vi "sinewave_generator_simulation_demoinfocom.vi"() -> ()   [LabVIEW 2021]
uses:
  <vilib>/addons/Modulation/Analog/controls/Complex Data Waveform.ctl
  <vilib>/Analysis/1siggen.llb/Ramp Pattern by Samples.vi
  system stop.vi
  <vilib>/measure/maspectr.llb/FFT Power Spectrum and PSD for 1 Chan (CDB).vi
  <vilib>/addons/Modulation/niAMT.lvlib
  <vilib>/Analysis/NI_AALBase.lvlib
  <vilib>/measure/NI_MAPro.lvlib
panel:
  out "Waveform Graph":cluster{"f0":dbl, "df":dbl, "magnitude":dbl[]}(graph)
  in  "Sampling Rate":dbl
  in  "duration":dbl
  in  "Frequency":dbl format="%#_13g"
  in  "stop":bool
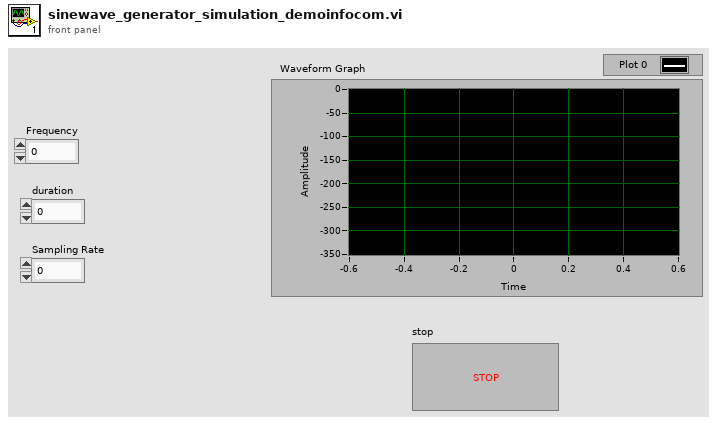
[diagram p1: front panel]
types:
  T1 = typedef "niAMT.lvlib/Complex Data Waveform.ctl" = cluster{"t0":dbl, "dt":dbl, "Y":cdb[]}
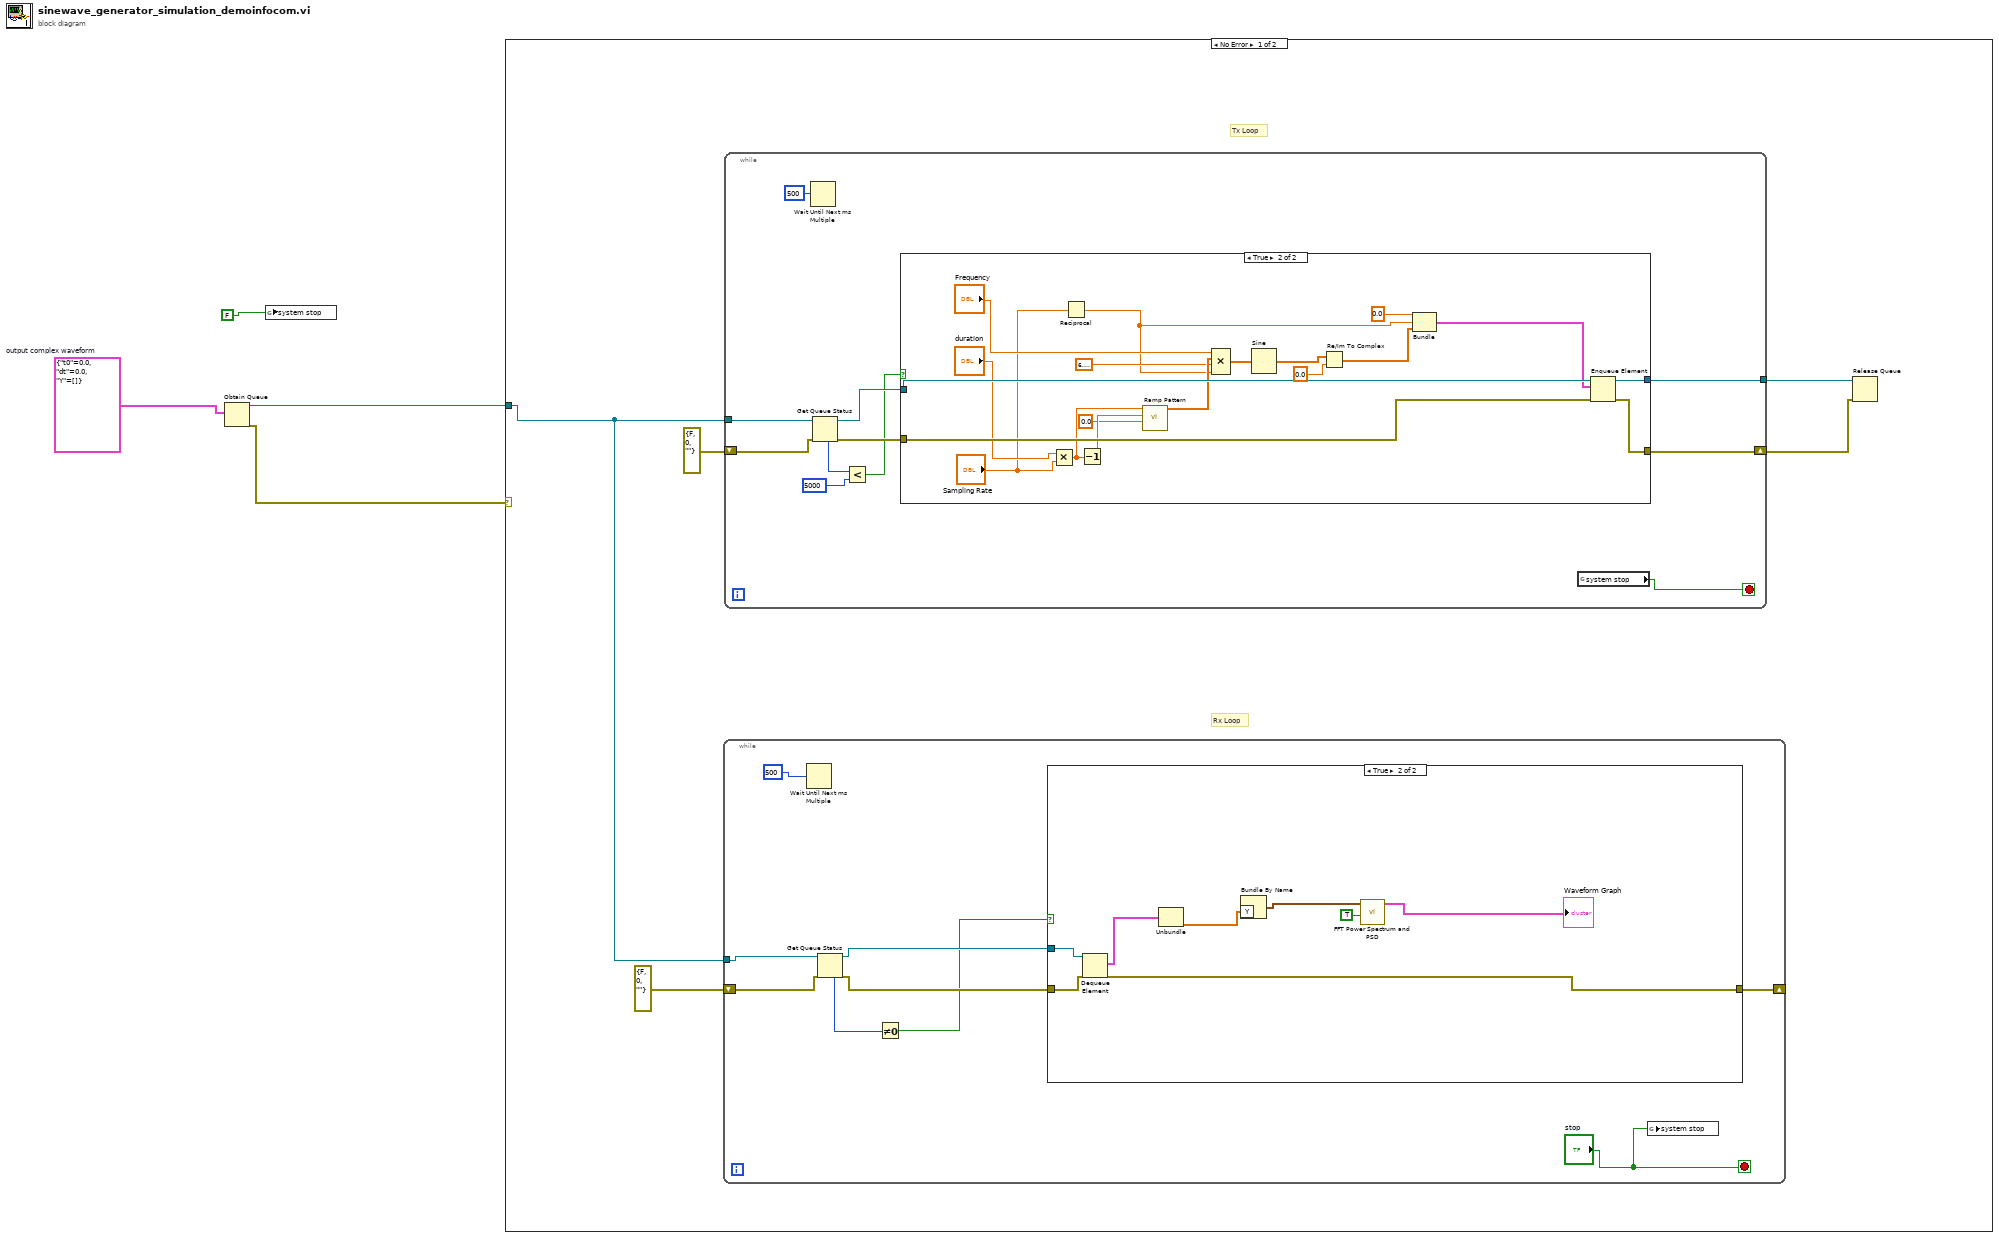
[diagram p0: block diagram]
diagram:
  w1 = T1 {"t0"=0.0, "dt"=0.0, "Y"=[]}  # output complex waveform
  n1 = Obtain Queue(element data type=w1) -> (queue out=w3:refnum<queue>, error out=w2:errorcluster)  [unwired: 4 in, 1 out]
  n2 = global write "system stop.vi" "system stop"(FALSE) -> ()
  n3 = case shown="No Error" w2 {
    tunnel: w3 -> [w8 _]
    frame No Error {
      # "Rx Loop"
      # "Tx Loop"
      n4 = while {
        tunnel: w8 -> [w17]
        shift-right: [w13] -> _
        shift-left: errorcluster {"status"=FALSE, "code"=0, "source"=""} ("error in (no error)") -> [w15]
        stop <- "stop" stop-if-true
        n5 = Wait Until Next ms Multiple(millisecond multiple=500) -> ()  [unwired: 1 out]
        n6 = Get Queue Status(queue=w17, error in (no error)=w15) -> (queue out=w16:refnum<queue>, error out=w14:errorcluster, # elements in queue=w12:i32)  [unwired: 1 in, 5 out]
        n7 = Not Equal To 0?(x=w12) -> (x != 0?=w11:bool)
        n8 = case shown="True" w11 {
          tunnel: w16 -> [_ w27]
          tunnel: w14 -> [w19 w26]
          tunnel: [w19 w25] -> w13
          frame False {
          }
          frame True {
            n9 = Dequeue Element(queue=w27, error in (no error)=w26) -> (element=w24:T1, error out=w25:errorcluster)  [unwired: 1 in, 2 out]
            n10 = Unbundle(w24) -> ("Y"=w23:cdb[])  [unwired: 2 out]
            n11 = Bundle By Name("Y"=w23) -> (w21:waveform(cdb))  [unwired: 1 in]
            n12 = call-poly <vilib>:"FFT Power Spectrum and PSD.vi"("dB On (F)"=TRUE, "time signal"=w21) -> ("Power Spectrum / PSD"=→"Waveform Graph":cluster{"f0":dbl, "df":dbl, "magnitude":dbl[]})  [unwired: 6 in, 3 out]
          }
        }
        n13 = global write "system stop.vi" "system stop"("stop") -> ()
      }
      n14 = while {
        tunnel: w8 -> [w37]
        shift-right: [w33] -> w5
        shift-left: errorcluster {"status"=FALSE, "code"=0, "source"=""} ("error in (no error)") -> [w36]
        tunnel: [w29] -> w6
        stop <- w38 stop-if-true
        n15 = Wait Until Next ms Multiple(millisecond multiple=500) -> ()  [unwired: 1 out]
        n16 = Get Queue Status(queue=w37, error in (no error)=w36) -> (queue out=w35:refnum<queue>, error out=w34:errorcluster, # elements in queue=w32:i32)  [unwired: 1 in, 5 out]
        n17 = Less?(x=w32, y=5000) -> (x < y?=w30:bool)
        n18 = case shown="True" w30 {
          tunnel: w35 -> [w39 w59]
          tunnel: w34 -> [w40 w58]
          tunnel: [w40 w56] -> w33
          tunnel: [w39 w57] -> w29
          frame False {
          }
          frame True {
            n19 = Multiply(x="duration", y="Sampling Rate") -> (x*y=w52:dbl)
            n20 = Reciprocal(x="Sampling Rate") -> (1/x=w44:dbl)
            n21 = Decrement(x=w52) -> (x-1=w53:dbl)
            n22 = call-poly <vilib>:"Ramp Pattern.vi"("start"=0.0, "end"=w53, "samples"=w52) -> ("Ramp Pattern"=w50:dbl[])  [unwired: 7 in, 1 out]
            n23 = Compound Arithmetic op=MULTIPLY("Frequency", w50, 6.283185307179586, w44) -> (w47:dbl[])
            n24 = Sine(x=w47) -> (sin(x)=w46:dbl[])
            n25 = Re/Im To Complex(1:0.0, 2:w46) -> (0:w42:cdb[])
            n26 = Bundle(0.0, w44, w42) -> (w41:cluster{dbl, dbl, cdb[]})  [unwired: 1 in]
            n27 = Enqueue Element(queue=w59, element=w41, error in (no error)=w58) -> (queue out=w57:refnum<queue>, error out=w56:errorcluster)  [unwired: 1 in, 1 out]
          }
        }
        n28 = global read "system stop.vi" "system stop"() -> (w38:bool)
      }
      n29 = Release Queue(queue=w6, error in (no error)=w5) -> ()  [unwired: 1 in, 3 out]
    }
    frame Error {
    }
  }
